vi "8.4.-Momento h1.vi"(1 "n20/n02":dbl[](array[numeric])) -> (0 "M1":dbl)   [LabVIEW 2020]
panel:
  # "Visión Artificial - Momentos Invariantes de Hu\nDiego Cervantes Rodríguez\ndicer0.com"
  # "M1 = n20+n02"
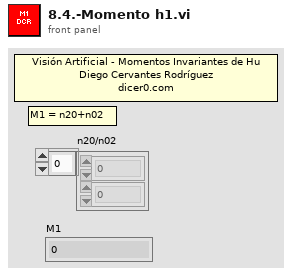
[diagram p1: front panel]
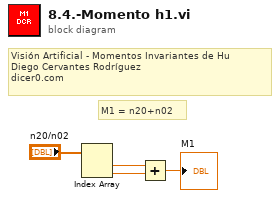
[diagram p0: block diagram]
diagram:
  # "Visión Artificial - Momentos Invariantes de Hu\nDiego Cervantes Rodríguez\ndicer0.com"
  # "M1 = n20+n02"
  n1 = Index Array "Index Array"(array="n20/n02") -> (element #1=w3:dbl, element #2=w2:dbl)  [unwired: 2 in]
  n2 = Add(x=w3, y=w2) -> (x+y=→"M1":dbl)
